vi "Plot_XY_data.vi"(0 "All Data In":string[][](array[string]), 1 "Ordinate Strings":string[](array[string]), 2 "Swap color and symbol":i32, 3 "Error bar ch index":T1[](array[typedef]), 5 "Accept Array":bool[][](array[boolean]), 9 "Colour Array":u32[][](array[colorbox])=[[26112, 39168, 52224, 65280, 65433], [153, 13311, 26367, 52479, 65535], [16711680, 16724838, 16737894, 16737945, 16751103], [16776960, 16777062, 16777113, 16777164, 16777215], [65280, 65280, 65280, 65280, 65280], [65280, 65280, 65280, 65280, 102]], 11 "Ordinate":i32[](array[numeric])=[11], 12 "Absisca":u16, 13 "Transpose":bool) -> (4 "X Scale.Format & Precision:Precision":u8, 15 "Accept Array Out":bool[][](array[boolean]))   [LabVIEW 2021]
uses:
  Error_bars_index.ctl
  Results_plotter_Global.vi
  Data plotting/subVIs/Plot_Values_Global.vi
panel:
  out "Point Choice":u8[](array[numeric])=[10, 1, 11, 15, 5, 13, 2, 14]
  in  "Index Filter2":i32
  in  "Index Filter1":i32
  in  "Index Ordinate":i32
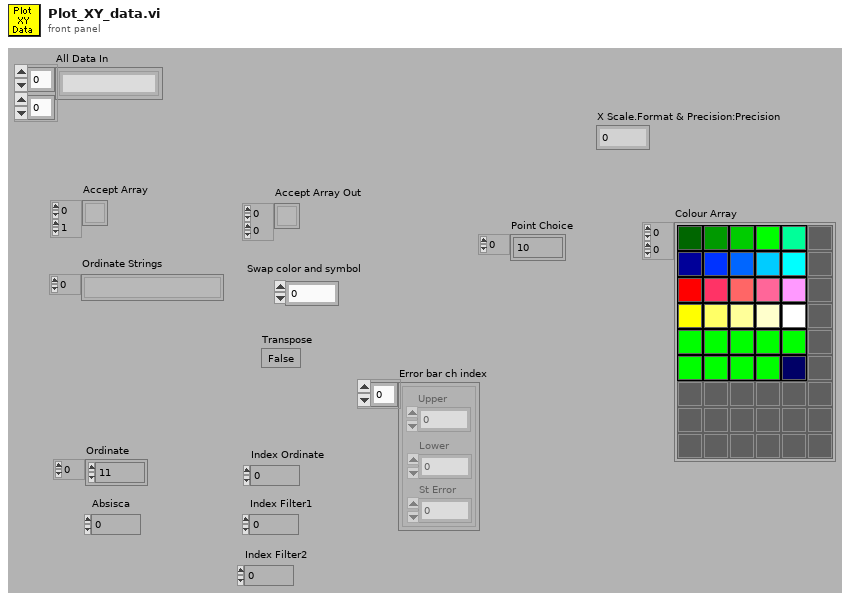
[diagram p1: front panel]
types:
  T1 = typedef "Error_bars_index.ctl" = cluster{"Upper":i32, "Lower":i32, "St Error":i32}
  T2 = cluster{"Plot Color":u32, "Plot Interpolation":u8, "Point Style":u8, "Line Style":u8, "Fill/Pt. Color":u32, "Line Width":u8, "Bar Plot Style":u8, "Fill To":i16}
  T3 = cluster{"Plot Color":u32, "Plot Interpolation":u8, "Point Style":u8, "Line Style":u8, "Fill/Pt. Color":u32, "Line Width":u8, "Bar Plot Style":u8, "Fill To":i16}[]
  T4 = typedef "RFP_Plot_Metadata.ctl" = cluster{"Row Number":i32[], "Error Bars":T1, "X Label":string, "Y Label":string, "Blanks NaNs":i32[]}
  T5 = cluster{"Positions out":dbl[], "Averaged Values":dbl[]}
  T6 = cluster{"Averaged Values":dbl[], "Positions out":dbl[]}
  T7 = cluster{"Averaged Values":dbl[], "Positions out":dbl[]}[]
  T8 = enum16{"Points", "StepLeft", "Line", "StepRight", "StepCentre", "StepEdge"}
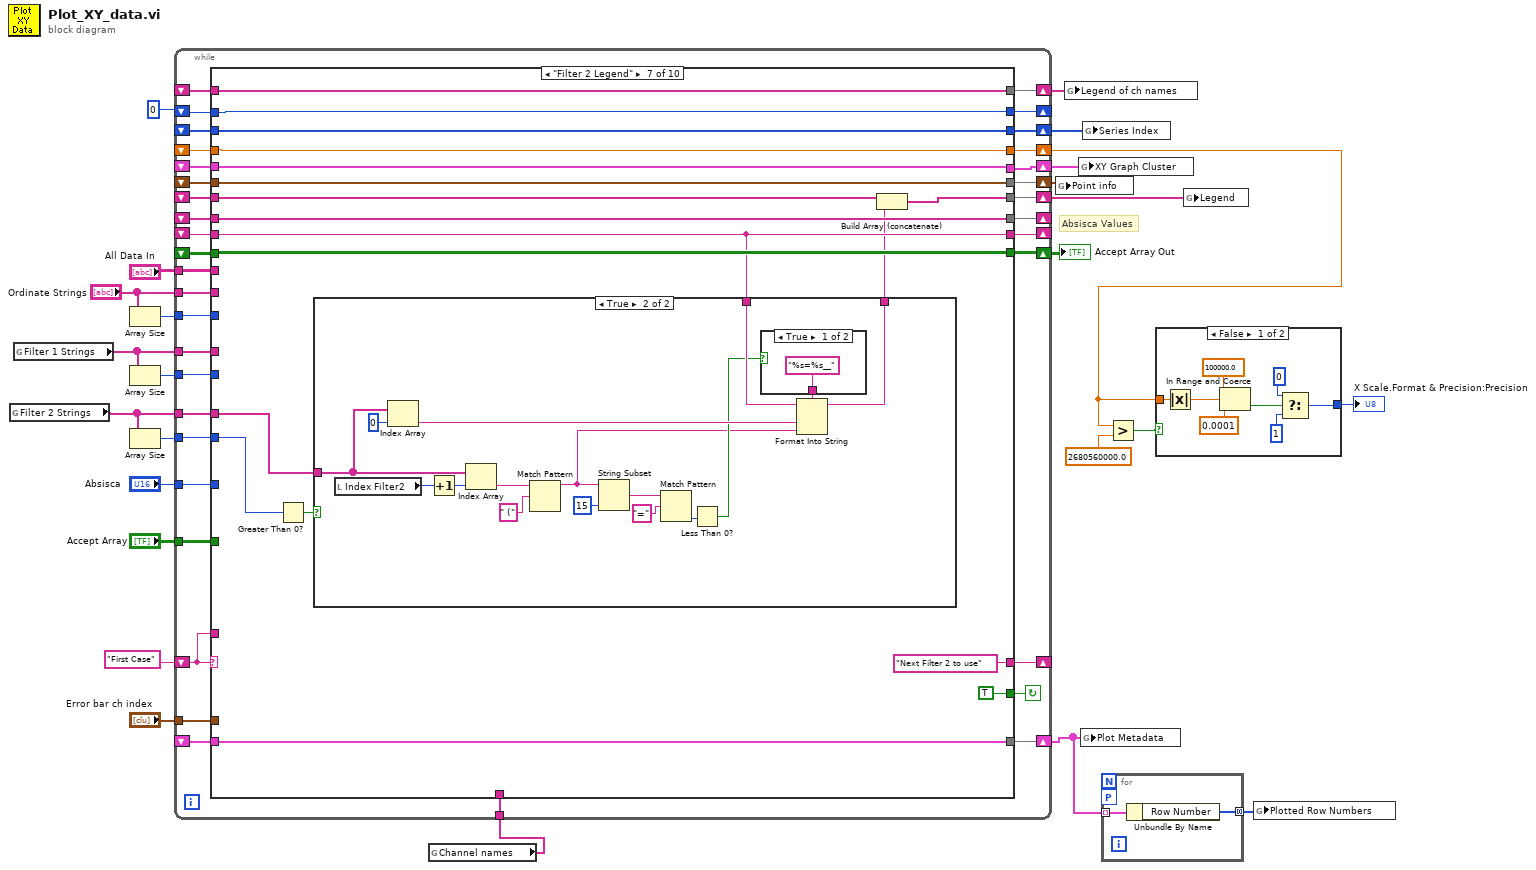
[diagram p0: block diagram]
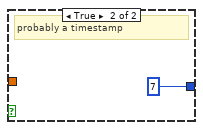
[diagram p2: hidden frame]
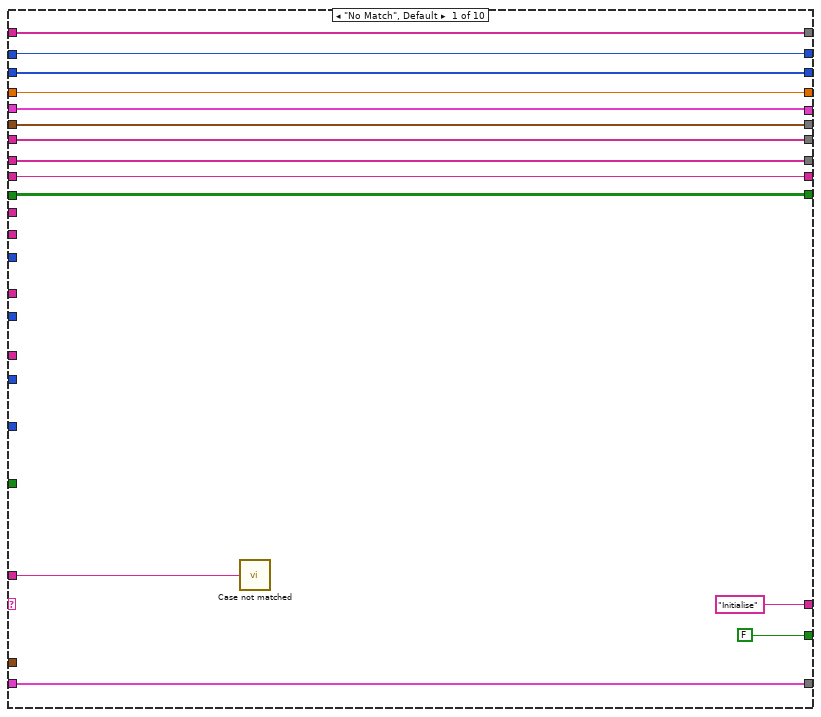
[diagram p3: hidden frame]
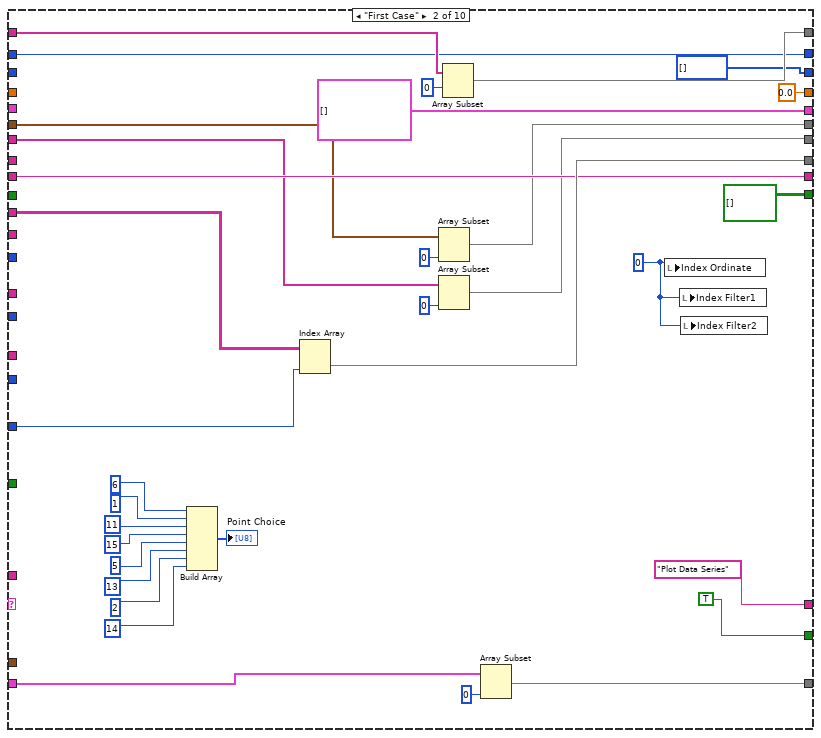
[diagram p4: hidden frame]
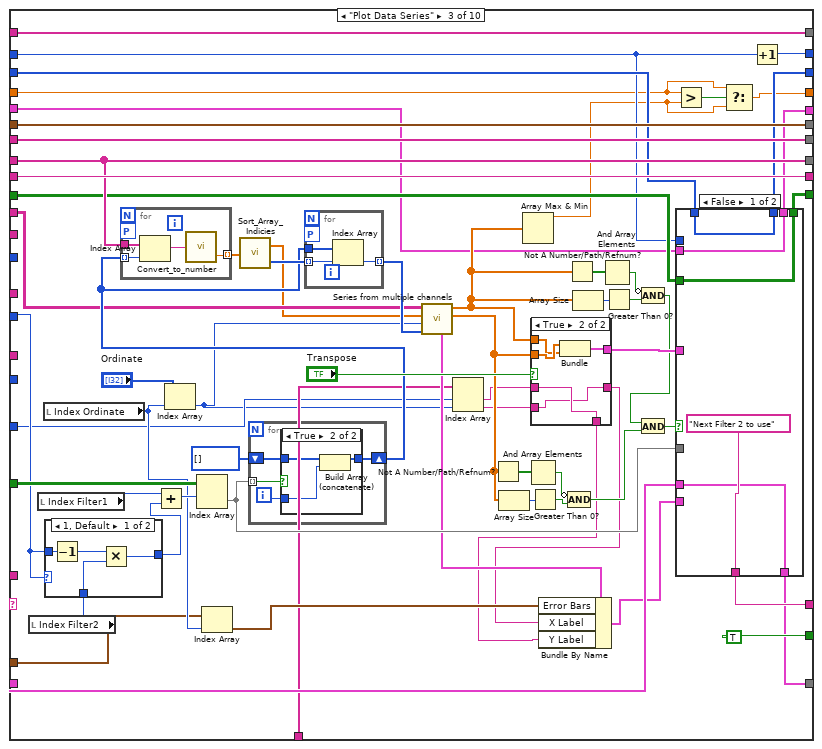
[diagram p5: hidden frame]
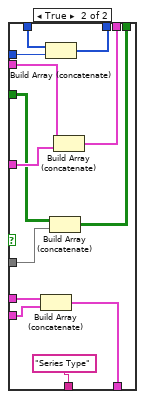
[diagram p7: hidden frame]
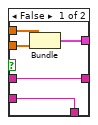
[diagram p8: hidden frame]
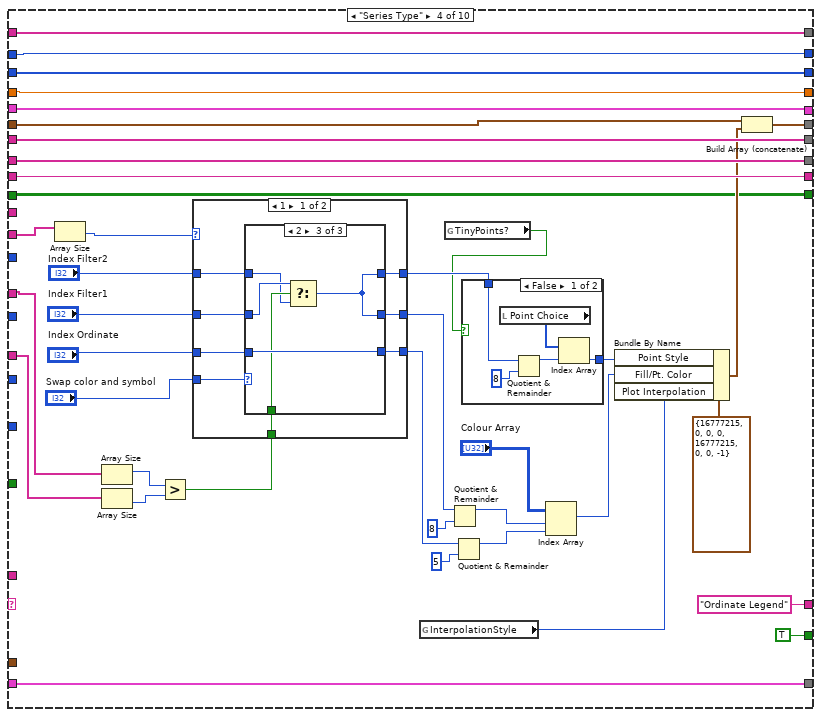
[diagram p10: hidden frame]
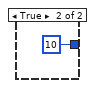
[diagram p11: hidden frame]
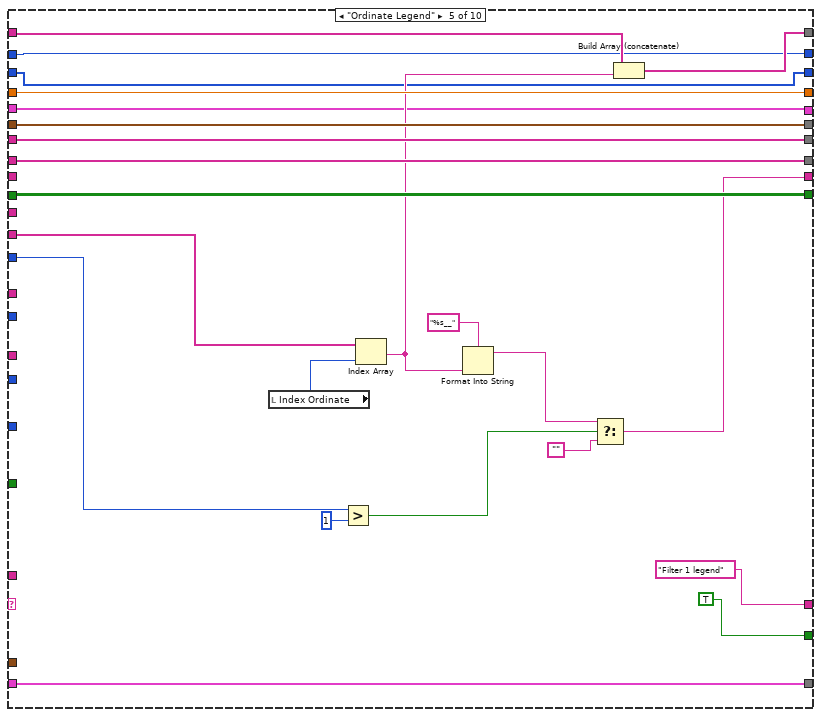
[diagram p20: hidden frame]
diagram:
  # "Absisca Values"
  n1 = global read "Results_plotter_Global.vi" "Filter 2 Strings"() -> (w11:string[])
  n2 = global read "Results_plotter_Global.vi" "Filter 1 Strings"() -> (w12:string[])
  n3 = Array Size(array="Ordinate Strings") -> (size(s)=w22:i32)
  n4 = Array Size(array=w12) -> (size(s)=w20:i32)
  n5 = Array Size(array=w11) -> (size(s)=w21:i32)
  n6 = global read "Results_plotter_Global.vi" "Channel names"() -> (w3:string[])
  n7 = while {
    shift-left: _ -> [w42]
    shift-right: [w41] -> w19
    tunnel: w20 -> [w43]
    tunnel: w21 -> [w44]
    tunnel: w22 -> [w45]
    tunnel: w12 -> [w46]
    tunnel: w11 -> [w47]
    tunnel: "Ordinate Strings" -> [w48]
    tunnel: "Accept Array" -> [w49]
    tunnel: "All Data In" -> [w50]
    shift-left: _ -> [w51]
    shift-right: [w52] -> _
    shift-left: _ -> [w53]
    shift-right: [w54] -> _
    shift-left: _ -> [w56]
    shift-right: [w55] -> w17
    shift-left: _ -> [w58]
    shift-right: [w57] -> w18
    shift-left: "First Case" -> [w59]
    shift-right: [w60] -> _
    shift-right: [w39] -> w5
    shift-left: _ -> [w40]
    shift-right: [w38] -> w16
    shift-left: _ -> [w37]
    tunnel: "Error bar ch index" -> [w36]
    shift-right: [w34] -> w10
    shift-left: _ -> [w35]
    shift-right: [w32] -> _
    shift-left: 0 -> [w33]
    shift-right: [w30] -> w14
    shift-left: _ -> [w31]
    tunnel: "Absisca" -> [w29]
    tunnel: w3 -> [w28]
    shift-right: [w27] -> w1
    shift-left: _ -> [w26]
    stop <- w61 continue-if-true
    n8 = case shown="\"Filter 2 Legend\"" w59 {
      tunnel: [FALSE TRUE TRUE TRUE TRUE TRUE TRUE TRUE TRUE w465] -> w61
      tunnel: ["Initialise" "Plot Data Series" w159 "Ordinate Legend" "Filter 1 legend" "Filter 2 Legend" "Next Filter 2 to use" w417 w441 w466] -> w60
      tunnel: w59 -> [w62 _ _ _ _ _ _ _ _ _]
      tunnel: w58 -> [w73 w91 w170 w249 w327 w344 w384 w426 w450 w475]
      tunnel: [w73 w90 w170 w247 w327 w344 w384 w426 w450 w475] -> w57
      tunnel: w56 -> [w72 w89 w169 w256 w329 w346 w381 w425 w449 w474]
      tunnel: [w72 w88 w169 w256 w329 w346 w382 w425 w449 w474] -> w55
      tunnel: [w71 w105 w166 w255 w328 w345 w385 w424 w448 w473] -> w54
      tunnel: w53 -> [w71 _ w166 w255 w328 w345 w385 w424 w448 w473]
      tunnel: [w70 w94 w168 w254 w316 w343 w374 w423 w447 w472] -> w52
      tunnel: w51 -> [w70 w94 w168 w254 _ w340 w374 w423 w447 w472]
      tunnel: w50 -> [_ w106 w129 _ _ _ _ _ _ _]
      tunnel: w49 -> [_ _ w165 _ _ _ _ _ _ _]
      tunnel: w48 -> [_ _ _ w235 w324 _ _ _ _ _]
      tunnel: w47 -> [_ _ _ w232 _ _ w372 _ _ _]
      tunnel: w46 -> [_ _ _ w233 _ w341 _ _ _ _]
      tunnel: w45 -> [_ _ _ _ w326 _ _ _ _ w463]
      tunnel: w44 -> [_ _ _ _ _ _ w383 w413 _ _]
      tunnel: w43 -> [_ _ w152 _ _ w339 _ _ w437 _]
      tunnel: w42 -> [w69 _ w157 w245 w323 w338 w380 w416 w440 w464]
      tunnel: [w69 bool[][] [] w155 w245 w323 w338 w380 w416 w440 w464] -> w41
      tunnel: w40 -> [w68 _ w120 w244 w322 w337 w379 w415 w439 w462]
      tunnel: [w68 0.0 w118 w244 w322 w337 w379 w415 w439 w462] -> w39
      tunnel: w37 -> [w67 w86 w151 w227 w313 w336 w378 w414 w438 w461]
      tunnel: [w67 w81 w151 w227 w314 w336 w378 w414 w438 w461] -> w38
      tunnel: w36 -> [_ _ w149 _ _ _ _ _ _ _]
      tunnel: w35 -> [w66 w83 w127 w226 w312 w335 w377 w412 w436 w460]
      tunnel: [w66 w82 w126 w226 w312 w335 w377 w412 w436 w460] -> w34
      tunnel: w33 -> [w65 w80 w132 w225 w311 w334 w376 w411 w435 w459]
      tunnel: [w65 w80 w135 w225 w311 w334 w376 w411 w435 w459] -> w32
      tunnel: w31 -> [w64 _ w134 w224 w310 w333 w375 w410 w434 w458]
      tunnel: [w64 i32[] [] w133 w224 w310 w333 w375 w410 w434 w458] -> w30
      tunnel: w29 -> [_ w77 w116 _ _ _ _ _ _ _]
      tunnel: w28 -> [_ _ w117 _ _ _ _ _ _ _]
      tunnel: [w63 cluster{dbl[], dbl[]}[] [] ("XY Graph Cluster In") w110 w221 w309 w332 w370 w409 w433 w457] -> w27
      tunnel: w26 -> [w63 _ w109 w221 w309 w332 w370 w409 w433 w457]
      frame "No Match", Default {
        n9 = call "Case not matched.vi"("Case Name not Matched"=w62) -> ()
      }
      frame "First Case" {
        w104 = 0
        n10 = Build Array(u8 6 ("Write Attribute"), u8 1 ("Write Attribute"), u8 11 ("Write Attribute"), u8 15 ("Write Attribute"), u8 5 ("Write Attribute"), u8 13 ("Write Attribute"), u8 2 ("Write Attribute"), u8 14 ("Write Attribute")) -> (→"Point Choice":u8[])
        n11 = Index Array(array=w106, index (col)=w77) -> (element=w105:string[])  [unwired: 1 in]
        n12 = Array Subset(array=w91, length=0 ("Array Length")) -> (w90:T3)  [unwired: 1 in]
        n13 = Array Subset(array=w89, length=0 ("Array Length")) -> (w88:string[])  [unwired: 1 in]
        n14 = Array Subset(array=w86, length=0) -> (w81:string[])  [unwired: 1 in]
        n15 = Array Subset(array=w83, length=0 ("Array Length")) -> (w82:T4[])  [unwired: 1 in]
        n16 = local write "Index Ordinate"(w104) -> ()
        n17 = local write "Index Filter1"(w104) -> ()
        n18 = local write "Index Filter2"(w104) -> ()
      }
      frame "Plot Data Series" {
        n19 = local read "Index Filter2"() -> (w154:i32)
        n20 = local read "Index Filter1"() -> (w164:i32)
        n21 = local read "Index Ordinate"() -> (w150:i32)
        n22 = case shown="1, Default" w152 {
          tunnel: w154 -> [w178 w179]
          tunnel: w152 -> [w177 _]
          tunnel: [w176 w179] -> w153
          frame 1, Default {
            n23 = Decrement(x=w177) -> (x-1=w175:i32)
            n24 = Multiply(x=w175, y=w178) -> (x*y=w176:i32)
          }
          frame 0 {
          }
        }
        n25 = Add(x=w164, y=w153) -> (x+y=w163:i32)
        n26 = Index Array(array="Ordinate", index=w150) -> (element=w115:i32)
        n27 = Index Array(array=w165, index (row)=w163) -> (element=w156:bool[])  [unwired: 1 in]
        n28 = Index Array(array=w149, index=w150) -> (element=w124:T1)
        n29 = for {
          shift-right: [w213] -> w146
          shift-left: i32[] [] -> [w214]
          tunnel: w156 -> [w212] mode=indexing
          i -> [w215]
          n30 = case shown="True" w212 {
            tunnel: w215 -> [_ w219]
            tunnel: w214 -> [w216 w218]
            tunnel: [w216 w217] -> w213
            frame False {
            }
            frame True {
              n31 = Build Array (concatenate)(w218, w219) -> (w217:i32[])
            }
          }
        }
        n32 = for {
          tunnel: w166 -> [w201]
          tunnel: [w199] -> w148 mode=indexing
          tunnel: w146 -> [w200] mode=indexing
          workers-P: _ -> [_]
          n33 = Index Array(array=w201, index=w200) -> (element=w198:string)
          n34 = call "Convert_to_number.vi"("string"=w198) -> ("Number"=w199:dbl)  [unwired: 1 out]
        }
        n35 = call "Sort_Array_Indicies.vi"("unsorted array"=w148) -> ("sorted array"=w128:dbl[], "Sort Index"=w147:i32[])
        n36 = for {
          tunnel: w147 -> [w174] mode=indexing
          tunnel: w146 -> [w173]
          tunnel: [w172] -> w131 mode=indexing
          workers-P: _ -> [_]
          n37 = Index Array(array=w173, index=w174) -> (element=w172:i32)
        }
        n38 = call "Series from multiple channels.vi"("Row Numbers"=w131, "Ordinate Index"=w115, "Positions In"=w128, "Channel Values"=w129) -> ("Averaged Values"=w130:dbl[], "Positions out"=w122:dbl[], "Plot Metadata"=w125:T4)  [unwired: 3 in, 2 out]
        n39 = Index Array(array=w117, index #1=w116, index #2=w115) -> (element #1=w114:string, element #2=w111:string)
        n40 = Not A Number/Path/Refnum?(number/path/refnum=w130) -> (NaN/Path/Refnum?=w141:bool[])
        n41 = Array Size(array=w130) -> (size(s)=w142:i32)
        n42 = Array Max & Min(array=w122) -> (max value=w119:dbl)  [unwired: 3 out]
        n43 = And Array Elements(Boolean array=w141) -> (logical AND=w139:bool)
        n44 = Greater Than 0?(x=w142) -> (x > 0?=w140:bool)
        n45 = case shown="True" "Transpose" {
          tunnel: w122 -> [w206 w209]
          tunnel: [w205 w211] -> w160
          tunnel: w130 -> [w204 w210]
          tunnel: w114 -> [w203 w208]
          tunnel: [w203 w207] -> w113
          tunnel: [w202 w208] -> w112
          tunnel: w111 -> [w202 w207]
          frame False {
            n46 = Bundle("Positions out"=w206, "Averaged Values"=w204) -> (w205:T5)  [unwired: 1 out]
          }
          frame True {
            n47 = Bundle("Averaged Values"=w210, "Positions out"=w209) -> (w211:T6)  [unwired: 1 out]
          }
        }
        n48 = Bundle By Name(cluster=w125, "Error Bars"=w124, "X Label"=w113, "Y Label"=w112) -> (w123:T4)
        n49 = Not A Number/Path/Refnum?(number/path/refnum=w122) -> (NaN/Path/Refnum?=w145:bool[])
        n50 = Compound Arithmetic op=AND(invert w139, w140) -> (w136:bool)
        n51 = Array Size(array=w122) -> (size(s)=w161:i32)
        n52 = And Array Elements(Boolean array=w145) -> (logical AND=w143:bool)
        n53 = Greater Than 0?(x=w161) -> (x > 0?=w144:bool)
        n54 = Compound Arithmetic op=AND(invert w143, w144) -> (w137:bool)
        n55 = And(x=w137, y=w136) -> (x .and. y?=w138:bool)
        n56 = Greater?(x=w120, y=w119) -> (0:w121:bool)
        n57 = case shown="False" w138 {
          tunnel: w160 -> [_ w197]
          tunnel: ["Next Filter 2 to use" "Series Type"] -> w159
          tunnel: w157 -> [w183 w195]
          tunnel: w156 -> [_ w194]
          tunnel: [w183 w193] -> w155
          tunnel: w134 -> [w182 w192]
          tunnel: [w182 w191] -> w133
          tunnel: w132 -> [_ w190]
          tunnel: w127 -> [w181 w189]
          tunnel: [w181 w188] -> w126
          tunnel: w123 -> [_ w187]
          tunnel: [w180 w186] -> w110
          tunnel: w109 -> [w180 w185]
          frame False {
          }
          frame True {
            n58 = Build Array (concatenate)(w189, w187) -> (w188:T4[])
            n59 = Build Array (concatenate)(w192, w190) -> (w191:i32[])
            n60 = Build Array (concatenate)(w195, w194) -> (w193:bool[][])
            n61 = Build Array (concatenate)(w185, w197) -> (w186:T7)
          }
        }
        n62 = Select(t=w120, s=w121, f=w119) -> (s? t:f=w118:dbl)
        n63 = Increment(x=w132) -> (x+1=w135:i32)
      }
      frame "Series Type" {
        n64 = Array Size(array=w235) -> (size(s)=w234:i32)
        n65 = Array Size(array=w233) -> (size(s)=w231:i32)
        n66 = Array Size(array=w232) -> (size(s)=w230:i32)
        n67 = Greater?(x=w231, y=w230) -> (0:w229:bool)
        n68 = case shown="1" w234 {
          tunnel: [w272 w290] -> w228
          tunnel: "Index Filter2" -> [w271 w289]
          tunnel: [w270 w288] -> w240
          tunnel: "Index Filter1" -> [w269 w287]
          tunnel: "Index Ordinate" -> [w268 w286]
          tunnel: [w267 w285] -> w237
          tunnel: "Swap color and symbol" -> [w266 w284]
          tunnel: w229 -> [w265 _]
          frame 1 {
            n69 = case shown="2" w266 {
              tunnel: [w275 w277 w279] -> w272
              tunnel: w271 -> [w275 w276 w280]
              tunnel: [w274 w276 w279] -> w270
              tunnel: w269 -> [w274 w277 w281]
              tunnel: w268 -> [w273 w278 w283]
              tunnel: [w273 w278 w283] -> w267
              tunnel: w265 -> [_ _ w282]
              frame 0, Default {
              }
              frame 1 {
              }
              frame 2 {
                n70 = Select(t=w281, s=w282, f=w280) -> (s? t:f=w279:i32)
              }
            }
          }
          frame 2, Default {
            n71 = case shown="4" w284 {
              tunnel: [w293 w295 w297 w301 w305 w308] -> w290
              tunnel: w289 -> [w293 w294 w297 w300 w303 w307]
              tunnel: [w292 w294 w299 w302 w304 w307] -> w288
              tunnel: w287 -> [w292 w295 w298 w301 w304 w306]
              tunnel: w286 -> [w291 w296 w299 w302 w305 w308]
              tunnel: [w291 w296 w298 w300 w303 w306] -> w285
              frame 0, Default {
              }
              frame 1 {
              }
              frame 2 {
              }
              frame 3 {
              }
              frame 4 {
              }
              frame 5 {
              }
            }
          }
        }
        n72 = global read "Results_plotter_Global.vi" "InterpolationStyle"() -> (w222:T8)
        n73 = global read "Results_plotter_Global.vi" "TinyPoints?"() -> (w223:bool)
        n74 = Quotient & Remainder(x=w240, y=8) -> (x-y*floor(x/y)=w243:i32)  [unwired: 1 out]
        n75 = Quotient & Remainder(x=w237, y=5) -> (x-y*floor(x/y)=w242:i32)  [unwired: 1 out]
        n76 = case shown="False" w223 {
          tunnel: [w262 u8 10 ("Write Attribute")] -> w251
          tunnel: w228 -> [w260 _]
          frame False {
            n77 = local read "Point Choice"() -> (w263:u8[])
            n78 = Quotient & Remainder(x=w260, y=8) -> (x-y*floor(x/y)=w259:i32)  [unwired: 1 out]
            n79 = Index Array(array=w263, index=w259) -> (element=w262:u8)
          }
          frame True {
          }
        }
        n80 = Index Array(array="Colour Array", index (row)=w243, index (col)=w242) -> (element=w250:u32)
        n81 = Bundle By Name(cluster=T2 {"Plot Color"=16777215, "Plot Interpolation"=0, "Point Style"=0, "Line Style"=0, "Fill/Pt. Color"=16777215, "Line Width"=0, "Bar Plot Style"=0, "Fill To"=-1} ("Read Attribute"), "Point Style"=w251, "Fill/Pt. Color"=w250, "Plot Interpolation"=w222) -> (w248:T2)
        n82 = Build Array (concatenate)(w249, w248) -> (w247:T3)
      }
      frame "Ordinate Legend" {
        n83 = local read "Index Ordinate"() -> (w320:i32)
        n84 = Greater?(x=w326, y=1) -> (0:w319:bool)
        n85 = Index Array(array=w324, index=w320) -> (element=w315:string)
        n86 = Format Into String(format string="%s__" ("Format String"), w315) -> (resulting string=w318:string)  [unwired: 2 in, 1 out]
        n87 = Select(t=w318, s=w319, f="") -> (s? t:f=w316:string)
        n88 = Build Array (concatenate)(w313, w315) -> (w314:string[])
      }
      frame "Filter 1 legend" {
        n89 = Greater Than 0?(x=w339) -> (x > 0?=w342:bool)
        n90 = case shown="False" w342 {
          tunnel: [w349 w361] -> w343
          tunnel: w341 -> [_ w360]
          tunnel: w340 -> [w351 w363]
          frame False {
            n91 = Concatenate Strings(w351, "None" ("string")) -> (w349:string)
          }
          frame True {
            n92 = local read "Index Filter1"() -> (w365:i32)
            n93 = Index Array(array=w360, index=0 ("Index")) -> (element=w358:string)
            n94 = Increment(x=w365) -> (x+1=w359:i32)
            n95 = Index Array(array=w360, index=w359) -> (element=w364:string)
            n96 = Match Pattern(string=w364, regular expression=" (") -> (before substring=w354:string)  [unwired: 4 out]
            n97 = String Subset(string=w354, length (rest)=15 ("length (rest)")) -> (substring=w352:string)  [unwired: 1 in]
            n98 = Match Pattern(string=w352, regular expression="=") -> (offset past match=w356:i32)  [unwired: 1 in, 3 out]
            n99 = Less Than 0?(x=w356) -> (x < 0?=w355:bool)
            n100 = case shown="False" w355 {
              tunnel: ["%s=%s__" ("Format String") "%s %s__" ("Format String")] -> w362
              frame True {
              }
              frame False {
              }
            }
            n101 = Format Into String(format string=w362, initial string=w363, w358, w354) -> (resulting string=w361:string)  [unwired: 1 in, 1 out]
          }
        }
      }
      frame "Filter 2 Legend" {
        n102 = Greater Than 0?(x=w383) -> (x > 0?=w371:bool)
        n103 = case shown="True" w371 {
          tunnel: [w388 w401] -> w373
          tunnel: w372 -> [_ w400]
          tunnel: w374 -> [w389 w403]
          frame False {
            n104 = Concatenate Strings(w389, "None" ("string")) -> (w388:string)
          }
          frame True {
            n105 = local read "Index Filter2"() -> (w394:i32)
            n106 = Index Array(array=w400, index=0 ("Index")) -> (element=w398:string)
            n107 = Increment(x=w394) -> (x+1=w399:i32)
            n108 = Index Array(array=w400, index=w399) -> (element=w404:string)
            n109 = Match Pattern(string=w404, regular expression=" (") -> (before substring=w392:string)  [unwired: 4 out]
            n110 = String Subset(string=w392, length (rest)=15 ("length (rest)")) -> (substring=w391:string)  [unwired: 1 in]
            n111 = Match Pattern(string=w391, regular expression="=") -> (offset past match=w396:i32)  [unwired: 1 in, 3 out]
            n112 = Less Than 0?(x=w396) -> (x < 0?=w395:bool)
            n113 = case shown="True" w395 {
              tunnel: ["%s=%s__" ("Format String") "%s %s__" ("Format String")] -> w402
              frame True {
              }
              frame False {
              }
            }
            n114 = Format Into String(format string=w402, initial string=w403, w398, w392) -> (resulting string=w401:string)  [unwired: 1 in, 1 out]
          }
        }
        n115 = Build Array (concatenate)(w381, w373) -> (w382:string[])
      }
      frame "Next Filter 2 to use" {
        n116 = local read "Index Filter2"() -> (w419:i32)
        n117 = Add(x=w419, y=2 ("x")) -> (x+y=w422:i32)
        n118 = Less?(x=w422, y=w413) -> (x < y?=w421:bool)
        n119 = case shown="False" w421 {
          tunnel: w419 -> [_ w432]
          tunnel: [0 w431] -> w418
          tunnel: ["Next Filter 1 to use" "Plot Data Series"] -> w417
          frame False {
          }
          frame True {
            n120 = Increment(x=w432) -> (x+1=w431:i32)
          }
        }
        n121 = local write "Index Filter2"(w418) -> ()
      }
      frame "Next Filter 1 to use" {
        n122 = local read "Index Filter1"() -> (w443:i32)
        n123 = Add(x=w443, y=2 ("x")) -> (x+y=w446:i32)
        n124 = Less?(x=w446, y=w437) -> (x < y?=w445:bool)
        n125 = case shown="True" w445 {
          tunnel: w443 -> [_ w456]
          tunnel: [0 w455] -> w442
          tunnel: ["Next Ordinate" "Plot Data Series"] -> w441
          frame False {
          }
          frame True {
            n126 = Increment(x=w456) -> (x+1=w455:i32)
          }
        }
        n127 = local write "Index Filter1"(w442) -> ()
      }
      frame "Next Ordinate" {
        n128 = local read "Index Ordinate"() -> (w468:i32)
        n129 = Add(x=w468, y=1 ("x")) -> (x+y=w471:i32)
        n130 = Less?(x=w471, y=w463) -> (x < y?=w470:bool)
        n131 = case shown="False" w470 {
          tunnel: w468 -> [_ w482]
          tunnel: [0 w481] -> w467
          tunnel: ["End" "Plot Data Series"] -> w466
          tunnel: [FALSE TRUE] -> w465
          frame False {
          }
          frame True {
            n132 = Increment(x=w482) -> (x+1=w481:i32)
          }
        }
        n133 = local write "Index Ordinate"(w467) -> ()
      }
    }
  }
  "Accept Array Out" <- w19
  n134 = global write "Results_plotter_Global.vi" "Point info"(w18) -> ()
  n135 = global write "Results_plotter_Global.vi" "Legend of ch names"(w16) -> ()
  n136 = global write "Plot_Values_Global.vi" "XY Graph Cluster"(w1) -> ()
  n137 = global write "Results_plotter_Global.vi" "Plot Metadata"(w10) -> ()
  n138 = global write "Results_plotter_Global.vi" "Series Index"(w14) -> ()
  n139 = for {
    tunnel: w10 -> [w484] mode=indexing
    tunnel: [w483] -> w9 mode=concatenating
    workers-P: _ -> [_]
    n140 = Unbundle By Name(w484) -> ("Row Number"=w483:i32[])
  }
  n141 = Greater?(x=w5, y=2680560000.0) -> (0:w7:bool)
  n142 = case shown="False" w7 {
    tunnel: [w486 u8 7 ("X Scale.Format & Precision:Precision")] -> w6
    tunnel: w5 -> [w492 _]
    frame False {
      n143 = Absolute Value(x=w492) -> (abs(x)=w485:dbl)
      n144 = In Range and Coerce(upper limit=100000.0 ("y"), x=w485, lower limit=0.0001) -> (In Range?=w489:bool)  [unwired: 1 out]
      n145 = Select(t=u8 0 ("f"), s=w489, f=u8 1) -> (s? t:f=w486:u8)
    }
    frame True {
      # "probably a timestamp"
    }
  }
  "X Scale.Format & Precision:Precision" <- w6
  n146 = global write "Results_plotter_Global.vi" "Legend"(w17) -> ()
  n147 = global write "Results_plotter_Global.vi" "Plotted Row Numbers"(w9) -> ()
